vi "BRig_dataTrial_I_anySelect_L.vi"() -> (2 "output_I_allReward_L":i32)   [LabVIEW 2014]
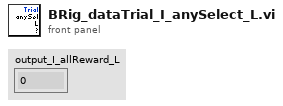
[diagram p1: front panel]
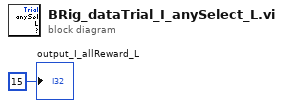
[diagram p0: block diagram]
diagram:
  "output_I_allReward_L" <- 15 ("output_iBlock")
